vi "incertezza_composta.vi"(8 "Descending uncertainty point-by-point":dbl[](array[numeric]), 11 "Ascending uncertainty point-by-point":dbl[](array[numeric])) -> (2 "incertezza_composta":dbl, 6 "ascending_uncertainty (absolute value)":dbl, 7 "descending_uncertainty (absolute value)":dbl)   [LabVIEW 2021]
uses:
  <vilib>/Analysis/baseanly.llb/Mean (DBL).vi
  <vilib>/Analysis/NI_AALBase.lvlib
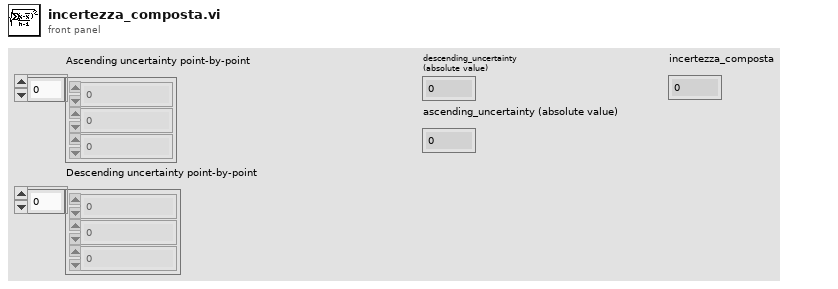
[diagram p1: front panel]
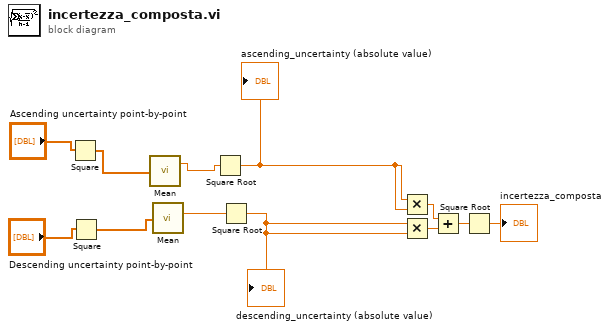
[diagram p0: block diagram]
diagram:
  n1 = Square(x="Ascending uncertainty point-by-point") -> (x^2=w10:dbl[])
  n2 = Square(x="Descending uncertainty point-by-point") -> (x^2=w9:dbl[])
  n3 = call-poly <vilib>:"Mean.vi"("X"=w10) -> ("mean"=w8:dbl)  [unwired: 1 out]
  n4 = call-poly <vilib>:"Mean.vi"("X"=w9) -> ("mean"=w7:dbl)  [unwired: 1 out]
  n5 = Square Root(x=w8) -> (sqrt(x)=w6:dbl)
  "ascending_uncertainty (absolute value)" <- w6
  n6 = Square Root(x=w7) -> (sqrt(x)=w5:dbl)
  "descending_uncertainty (absolute value)" <- w5
  n7 = Multiply(x=w6, y=w6) -> (x*y=w3:dbl)
  n8 = Multiply(x=w5, y=w5) -> (x*y=w2:dbl)
  n9 = Add(x=w3, y=w2) -> (x+y=w1:dbl)
  n10 = Square Root(x=w1) -> (sqrt(x)=→"incertezza_composta":dbl)
